vi "Websocket_CleanUp.vi"(5 "error in (no error)":errorcluster) -> (19 "error out":errorcluster)   [LabVIEW 2014, in "FrontPanelPublisher.lvlib" / "Websocket.lvclass"]
uses:
  Websocket.lvclass
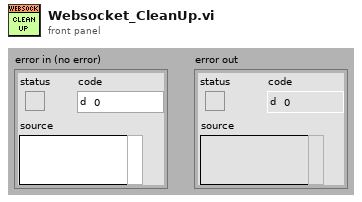
[diagram p1: front panel]
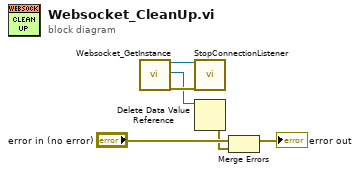
[diagram p0: block diagram]
diagram:
  n1 = call "Websocket_GetInstance.vi"() -> ("reference out"=w2:refnum<class "Websocket.lvclass">, "DVRRefOut"=w1:refnum<data-value>, "error out"=w3:errorcluster)  [unwired: 15 in, 2 out]
  n2 = call "StopConnectionListener.vi"("reference in"=w2, "error in (no error)"=w3) -> ()  [unwired: 16 in, 2 out]
  n3 = Delete Data Value Reference(data value reference=w1) -> (error out=w4:errorcluster)  [unwired: 1 in, 1 out]
  n4 = Merge Errors("error in (no error)", w4) -> (→"error out":errorcluster)
